vi "원격제어 대상.vi"() -> ()   [LabVIEW 2014]
uses:
  <vilib>/Utility/sysdir.llb/System Directory Type.ctl
panel:
  out "standard output 2":string caption="표준 출력"
  out "W":string
  out "D":string
  out "A":string
  out "S":string
  out "스페이스바":string
  out "스페이스바  2":string
  out "스페이스바3":string
  out "key의숫자값":i16[](array[numeric])
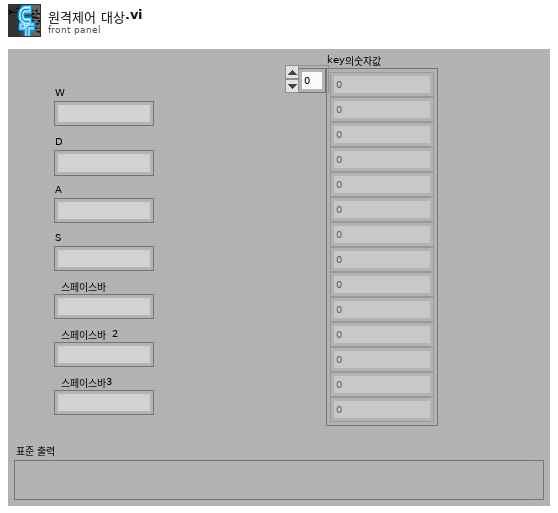
[diagram p1: front panel]
types:
  T1 = enum16{"open", "replace", "create", "open or create", "replace or create", "replace or create with confirmation"}
  T2 = typedef "System Directory Type.ctl" = i32
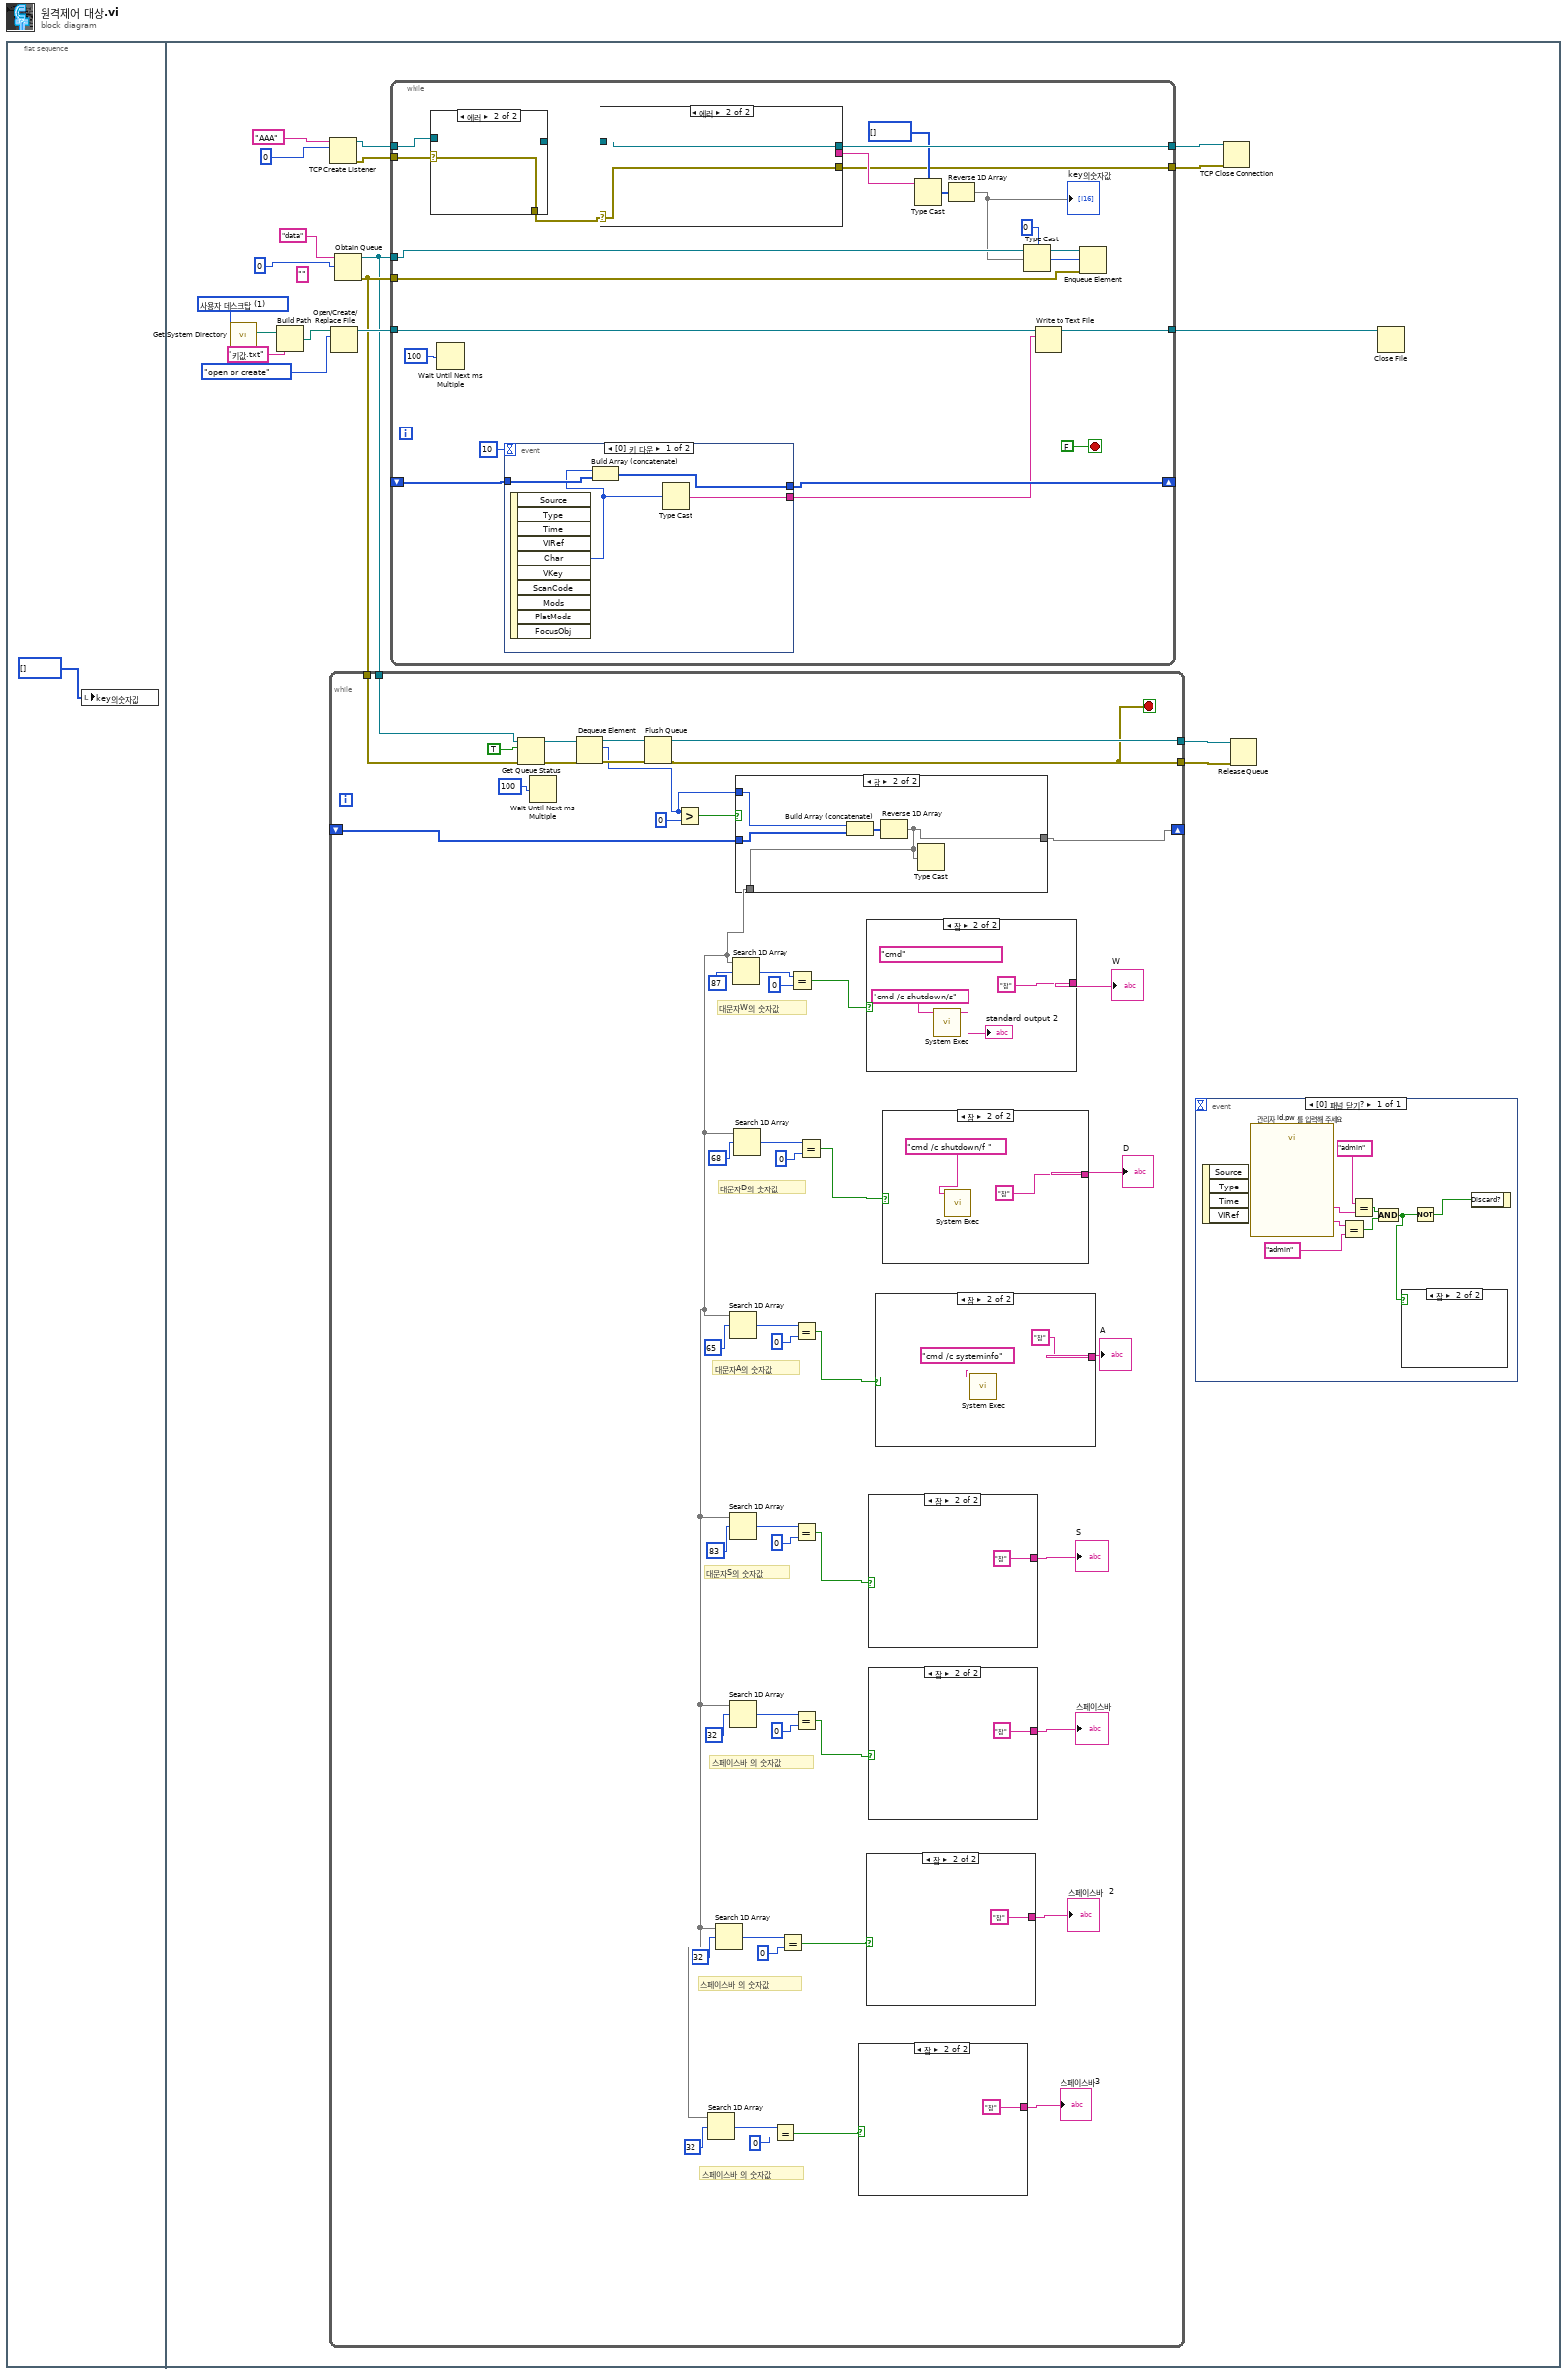
[diagram p0: block diagram]
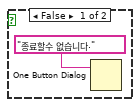
[diagram p2: hidden frame]
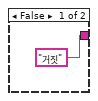
[diagram p4: hidden frame]
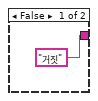
[diagram p5: hidden frame]
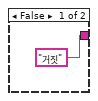
[diagram p6: hidden frame]
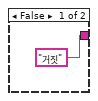
[diagram p7: hidden frame]
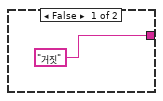
[diagram p8: hidden frame]
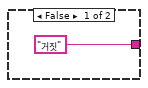
[diagram p9: hidden frame]
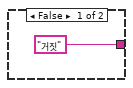
[diagram p10: hidden frame]
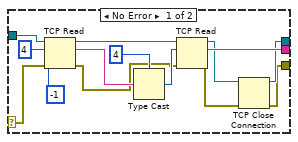
[diagram p11: hidden frame]
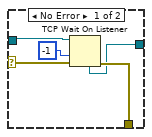
[diagram p12: hidden frame]
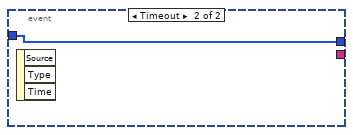
[diagram p13: hidden frame]
diagram:
  n1 = flat-sequence {
    frame #0 {
      n2 = local write "key의숫자값"(i16[] []) -> ()
    }
    frame #1 {
      (unwired) ""
      w18 = T2 1 items=["사용자 홈"=0, "사용자 데스크탑"=1, "사용자 문서"=2, "사용자 어플리케이션 데이터"=3, "사용자 환경"=4, "사용자 임시"=5, "퍼블릭 문서"=6, "퍼블릭 어플리케이션 데이터"=7, "퍼블릭 환경"=8, "퍼블릭 캐시"=13, "시스템 코어 라이브러리"=9, "시스템 설치된 라이브러리"=10, "어플리케이션 파일"=11, "부팅 볼륨 루트"=12] ("system directory type")
      n3 = call <vilib>:"Get System Directory.vi"("system directory type"=w18) -> ("system directory"=w17:path)  [unwired: 10 in]
      n4 = Build Path(base path=w17, name or relative path="키값.txt" ("이름 또는 상대 경로")) -> (appended path=w14:path)
      n5 = TCP Create Listener(10:u16 0 ("포트"), 11:"AAA" ("서비스 이름")) -> (0:w3:errorcluster, 3:w6:refnum<k5>)  [unwired: 1 in, 3 out]
      n6 = Open/Create/Replace File(file path (use dialog)=w14, operation (0:open)=T1."open or create" ("동작(0:open)")) -> (refnum out=w13:refnum<file>)  [unwired: 4 in, 2 out]
      n7 = Obtain Queue(name (unnamed)="data" ("이름(이름없음)"), element data type=i16 0) -> (queue out=w7:refnum<queue>, error out=w8:errorcluster)  [unwired: 3 in, 1 out]
      n8 = while {
        shift-right: [w41] -> _
        shift-left: _ -> [w42]
        tunnel: [w33] -> w10
        tunnel: [w32] -> w9
        tunnel: w7 -> [w39]
        tunnel: w8 -> [w38]
        stop <- w32 stop-if-true
        # "스페이스바 의 숫자값"
        # "스페이스바 의 숫자값"
        # "대문자W의 숫자값"
        # "대문자D의 숫자값"
        # "대문자A의 숫자값"
        # "대문자S의 숫자값"
        # "스페이스바 의 숫자값"
        n9 = Get Queue Status(queue=w39, return elements? (F)=TRUE ("원소 반환? (거짓)"), error in (no error)=w38) -> (queue out=w37:refnum<queue>, error out=w36:errorcluster)  [unwired: 6 out]
        n10 = Wait Until Next ms Multiple(millisecond multiple=u32 100) -> ()  [unwired: 1 out]
        n11 = Dequeue Element(queue=w37, error in (no error)=w36) -> (queue out=w34:refnum<queue>, element=w30:i16, error out=w35:errorcluster)  [unwired: 1 in, 1 out]
        n12 = Flush Queue(queue=w34, error in (no error)=w35) -> (queue out=w33:refnum<queue>, error out=w32:errorcluster)  [unwired: 1 out]
        n13 = Greater?(x=w30, y=i16 0) -> (0:w31:bool)
        n14 = case shown="참" w31 {
          tunnel: w42 -> [w81 w85]
          tunnel: w30 -> [_ w84]
          tunnel: [w81 w82] -> w41
          tunnel: [_ w82] -> w40
          frame False {
          }
          frame True {
            n15 = Build Array (concatenate)(w84, w85) -> (w83:i16[])
            n16 = Reverse 1D Array(array=w83) -> (reversed array=w82:i16[])
            n17 = Type Cast(x=w82) -> ()  [unwired: 1 in, 1 out]
          }
        }
        n18 = Search 1D Array(1D array=w40, element=i16 32 ("원소")) -> (index of element=w48:i32)  [unwired: 1 in]
        n19 = Search 1D Array(1D array=w40, element=i16 32 ("원소")) -> (index of element=w53:i32)  [unwired: 1 in]
        n20 = Search 1D Array(1D array=w40, element=i16 65 ("원소")) -> (index of element=w68:i32)  [unwired: 1 in]
        n21 = Search 1D Array(1D array=w40, element=i16 83 ("원소")) -> (index of element=w67:i32)  [unwired: 1 in]
        n22 = Search 1D Array(1D array=w40, element=i16 32 ("원소")) -> (index of element=w60:i32)  [unwired: 1 in]
        n23 = Search 1D Array(1D array=w40, element=i16 87 ("원소")) -> (index of element=w78:i32)  [unwired: 1 in]
        n24 = Search 1D Array(1D array=w40, element=i16 68 ("원소")) -> (index of element=w76:i32)  [unwired: 1 in]
        n25 = Equal?(x=w48, y=0) -> (x = y?=w50:bool)
        n26 = Equal?(x=w53, y=0) -> (x = y?=w51:bool)
        n27 = Equal?(x=w78, y=0) -> (x = y?=w75:bool)
        n28 = Equal?(x=w68, y=0) -> (x = y?=w70:bool)
        n29 = Equal?(x=w67, y=0) -> (x = y?=w65:bool)
        n30 = Equal?(x=w60, y=0) -> (x = y?=w62:bool)
        n31 = Equal?(x=w76, y=0) -> (x = y?=w73:bool)
        n32 = case shown="참" w50 {
          tunnel: ["거짓" "참"] -> w46
          frame False {
          }
          frame True {
          }
        }
        "스페이스바3" <- w46
        n33 = case shown="참" w75 {
          tunnel: ["거짓" "참"] -> w80
          frame False {
          }
          frame True {
            (unwired) "cmd" ("command line")
            n34 = call <vilib>:"System Exec.vi"("command line"="cmd /c shutdown/s" ("standard input")) -> ("standard output"=→"standard output 2":string)  [unwired: 7 in, 3 out]
          }
        }
        "W" <- w80
        n35 = case shown="참" w51 {
          tunnel: ["거짓" "참"] -> w55
          frame False {
          }
          frame True {
          }
        }
        "스페이스바  2" <- w55
        n36 = case shown="참" w65 {
          tunnel: ["거짓" "참"] -> w66
          frame False {
          }
          frame True {
          }
        }
        "S" <- w66
        n37 = case shown="참" w62 {
          tunnel: ["거짓" "참"] -> w61
          frame False {
          }
          frame True {
          }
        }
        "스페이스바" <- w61
        n38 = case shown="참" w70 {
          tunnel: ["거짓" "참"] -> w69
          frame False {
          }
          frame True {
            n39 = call <vilib>:"System Exec.vi"("command line"="cmd /c systeminfo" ("standard input")) -> ()  [unwired: 7 in, 4 out]
          }
        }
        "A" <- w69
        n40 = case shown="참" w73 {
          tunnel: ["거짓" "참"] -> w74
          frame False {
          }
          frame True {
            n41 = call <vilib>:"System Exec.vi"("command line"="cmd /c shutdown/f " ("standard input")) -> ()  [unwired: 7 in, 4 out]
          }
        }
        "D" <- w74
      }
      n42 = while {
        tunnel: w6 -> [w107]
        tunnel: [w125] -> w20
        tunnel: w13 -> [w121]
        tunnel: [w122] -> w19
        tunnel: w7 -> [w120]
        tunnel: w8 -> [w119]
        shift-right: [w111] -> _
        shift-left: _ -> [w112]
        tunnel: w3 -> [w108]
        tunnel: [w106] -> w2
        stop <- FALSE stop-if-true
        n43 = case shown="에러" w108 {
          selector: w108 -> [w146 w147]
          tunnel: [w145 w147] -> w105
          tunnel: w107 -> [w144 _]
          tunnel: [w142 _] -> w104
          frame No Error {
            n44 = TCP Wait On Listener(8:w146, 9:-1 ("타임아웃 ms (계속 기다림: -1)"), 11:w144) -> (0:w145:errorcluster, 4:w142:refnum<k5>)  [unwired: 4 out]
          }
          frame Error {
          }
        }
        n45 = Wait Until Next ms Multiple(millisecond multiple=u32 100) -> ()  [unwired: 1 out]
        n46 = event shown="[0] 키 다운" {
          selector: _ -> [_ _]
          dyn-events: _ -> [_ _]
          timeout: 10 -> [_ _]
          tunnel: [w150 w152] -> w111
          tunnel: w112 -> [w151 w152]
          tunnel: [w148 _] -> w109
          event Key Down {
            n47 = event-data() -> ("Char"=w149:i16)  [unwired: 1 in, 9 out]
            n48 = Build Array (concatenate)(w149, w151) -> (w150:i16[])
            n49 = Type Cast(x=w149) -> (*(type *) &x=w148:string)  [unwired: 1 in]
          }
          event Timeout {
            n50 = event-data() -> ()  [unwired: 1 in, 3 out]
          }
        }
        n51 = case shown="에러" w105 {
          selector: w105 -> [w131 w141]
          tunnel: [w129 w140] -> w125
          tunnel: [w134 _] -> w118
          tunnel: [w127 w141] -> w106
          tunnel: w104 -> [w126 w140]
          frame No Error {
            n52 = TCP Read(connection ID=w126, bytes to read=4, error in (no error)=w131, 9:-1 ("타임아웃 ms (25000)")) -> (connection ID out=w137:refnum<k5>, data out=w139:string, error out=w132:errorcluster)  [unwired: 1 in]
            n53 = Type Cast(type=4 ("bytes to read"), x=w139) -> (*(type *) &x=w133:i32)
            n54 = TCP Read(connection ID=w137, bytes to read=w133, error in (no error)=w132) -> (connection ID out=w130:refnum<k5>, data out=w134:string, error out=w128:errorcluster)  [unwired: 2 in]
            n55 = TCP Close Connection(connection ID=w130, error in (no error)=w128) -> (connection ID out=w129:refnum<k5>, error out=w127:errorcluster)  [unwired: 1 out]
          }
          frame Error {
          }
        }
        n56 = Type Cast(type=i16[] [], x=w118) -> (*(type *) &x=w115:i16[])
        n57 = Reverse 1D Array(array=w115) -> (reversed array=w113:i16[])
        "key의숫자값" <- w113
        n58 = Type Cast(type=i16 0, x=w113) -> (*(type *) &x=w116:i16)
        n59 = Write to Text File(file (use dialog)=w121, text=w109) -> (refnum out=w122:refnum<file>)  [unwired: 2 in, 2 out]
        n60 = Enqueue Element(queue=w120, element=w116, error in (no error)=w119) -> ()  [unwired: 1 in, 3 out]
      }
      n61 = event shown="[0] 패널 닫기?" {
        selector: _ -> [_]
        dyn-events: _ -> [_]
        timeout: _ -> [_]
        event Panel Close? {
          n62 = event-data() -> ()  [unwired: 1 in, 4 out]
          n63 = call "관리자 id.pw 를 입력해 주세요"() -> ("PW"=w28:string, "ID"=w25:string)  [unwired: 16 in, 2 out]
          n64 = Equal?(x=w28, y="admin") -> (x = y?=w24:bool)
          n65 = Equal?(x="admin", y=w25) -> (x = y?=w23:bool)
          n66 = And(x=w23, y=w24) -> (x .and. y?=w21:bool)
          n67 = case shown="참" w21 {
            frame False {
              n68 = One Button Dialog(message="종료할수 없습니다." ("메시지")) -> ()  [unwired: 1 in, 1 out]
            }
            frame True {
            }
          }
          n69 = Not(x=w21) -> (.not. x?=w22:bool)
          n70 = event-data("Discard?"=w22) -> ()  [unwired: 1 in, 1 out]
        }
      }
      n71 = TCP Close Connection(connection ID=w20, error in (no error)=w2) -> ()  [unwired: 1 in, 2 out]
      n72 = Release Queue(queue=w10, error in (no error)=w9) -> ()  [unwired: 1 in, 3 out]
      n73 = Close File(refnum=w19) -> ()  [unwired: 1 in, 2 out]
    }
  }
